vi "Default Settings.vi"(8 "error in (no error)":errorcluster, 11 "Routine in":refnum<class "Routine.lvclass">) -> (0 "error out":errorcluster, 3 "Routine out":refnum<class "Routine.lvclass">)   [LabVIEW 2020, in "Routine.lvclass"]
uses:
  Routine.lvclass
panel:
  # "This Routine does not Accept Settings"
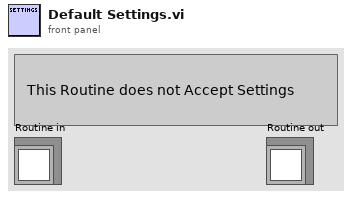
[diagram p1: front panel]
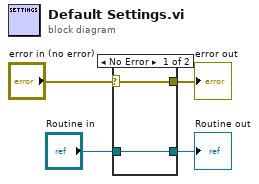
[diagram p0: block diagram]
diagram:
  n1 = case shown="No Error" "error in (no error)" {
    selector: "error in (no error)" -> [w5 w8]
    tunnel: [w5 w8] -> w3
    tunnel: [w6 w7] -> w1
    tunnel: "Routine in" -> [w6 w7]
    frame No Error {
    }
    frame Error {
    }
  }
  "error out" <- w3
  "Routine out" <- w1
